vi "HovaCAL set params konfig.vi"(8 "Fehler (Eingang, kein Fehler)":errorcluster, 10 "Pump Idx":i32, 11 "TestKonfig (Eingang)":T1 {"TestKonfig Interferent"."Gasflasche MFC3" items=["----"=10000, "IAG NH3 3000"=0, "IAG NH3 200"=1, "IAG NH3 2000"=2, "IAG MG"=3, "IAG O2"=4]; "TestKonfig Interferent"."Gasflasche MFC2" items=["----"=10000, "IAG NH3 3000"=0, "IAG NH3 200"=1, "IAG NH3 2000"=2, "IAG MG"=3, "IAG O2"=4]; "TestKonfig Interferent"."Eingangs Konzentration MFC1" min=0.0; "TestKonfig Interferent"."Ausgangs Konzentration MFC1" min=0.0; "TestKonfig Interferent"."MFC2" items=["MFC 2", "MFC 3", "MFC 4", "MFC 5"]; "TestKonfig Interferent"."MFC3" items=["MFC 2", "MFC 3", "MFC 4", "MFC 5"]; "TestKonfig Interferent"."Ausgangs Konzentration MFC3" min=0.0; "TestKonfig Interferent"."Eingangs Konzentration MFC3" min=0.0; "TestKonfig Interferent"."Ausgangs Konzentration MFC2" min=0.0; "TestKonfig Interferent"."Eingangs Konzentration MFC2" min=0.0; "TestKonfig H2O"."HovaCAL Temperature" format="%.2f"; "TestKonfig H2O"."HovaCAL Flow Input Cluster"."HovaCAL Flow Input Cluster" format="%.2f"; "TestKonfig H2O"."Eingangs Konzentration:" min=0.0; "TestKonfig H2O"."zusätzliche Zeitdauer Erster Punkt" min=30 step=1 format="%#_5g"; "TestKonfig H2O"."Zeitdauer Stufen" format="%#_5g"; "TestKonfig H2O"."Max Fehler" format="%#_5g"; "TestKonfig H2O"."Anzahl Stufen" format="%#_5g"; "TestKonfig H2O"."Modus" items=["Messen", "CG zu Entnahmestelle"]}) -> (0 "Fehler (Ausgang)":errorcluster, 3 "TestKonfig (Ausgang)":T1 {"TestKonfig Interferent"."Gasflasche MFC3" items=["----"=10000, "IAG NH3 3000"=0, "IAG NH3 200"=1, "IAG NH3 2000"=2, "IAG MG"=3, "IAG O2"=4]; "TestKonfig Interferent"."Gasflasche MFC2" items=["----"=10000, "IAG NH3 3000"=0, "IAG NH3 200"=1, "IAG NH3 2000"=2, "IAG MG"=3, "IAG O2"=4]; "TestKonfig Interferent"."Eingangs Konzentration MFC1" min=0.0; "TestKonfig Interferent"."Ausgangs Konzentration MFC1" min=0.0; "TestKonfig Interferent"."MFC2" items=["MFC 2", "MFC 3", "MFC 4", "MFC 5"]; "TestKonfig Interferent"."MFC3" items=["MFC 2", "MFC 3", "MFC 4", "MFC 5"]; "TestKonfig Interferent"."Ausgangs Konzentration MFC3" min=0.0; "TestKonfig Interferent"."Eingangs Konzentration MFC3" min=0.0; "TestKonfig Interferent"."Ausgangs Konzentration MFC2" min=0.0; "TestKonfig Interferent"."Eingangs Konzentration MFC2" min=0.0; "TestKonfig H2O"."HovaCAL Temperature" format="%.2f"; "TestKonfig H2O"."HovaCAL Flow Input Cluster"."HovaCAL Flow Input Cluster" format="%.2f"; "TestKonfig H2O"."Eingangs Konzentration:" min=0.0; "TestKonfig H2O"."zusätzliche Zeitdauer Erster Punkt" min=30 step=1 format="%#_5g"; "TestKonfig H2O"."Zeitdauer Stufen" format="%#_5g"; "TestKonfig H2O"."Max Fehler" format="%#_5g"; "TestKonfig H2O"."Anzahl Stufen" format="%#_5g"; "TestKonfig H2O"."Modus" items=["Messen", "CG zu Entnahmestelle"]})   [LabVIEW 2020, in "EPA 1065.lvlib" / "HovaCAL Interference verificaton.lvlib"]
uses:
  HovaCAL Interference verificaton.lvlib
  TestKonfig.ctl
  TestKonfig H2O.ctl
  Modus.ctl
  Linearisierung V2/SpanEinstellungen/Einheit.ctl
  Linearisierung V2/Gasteiler/Stufen Tabelle 10 Stufen.ctl
  Linearisierung V2/Gasteiler/HovaCAL_Interface/Controls/Flow Einstellung.ctl
  Linearisierung V2/Gasteiler/HovaCAL_Interface/Controls/Temp Sollwerte Anzeige.ctl
  TestKonfig Interferents.ctl
  MFCAuswahl.ctl
  Seiten/System Einstellungen V2/Gasflasche Auswahl.ctl
  Linearisierung V2/Gasteiler/HovaCAL_Interface/Kommunikation/Aktion_FGV_HovaCAL_Interface_Kommunikation.ctl
  Linearisierung V2/Gasteiler/HovaCAL_Interface/Kommunikation/Aktion_FGV_HovaCAL_Interface_Kommandos.ctl
  Aktion Index uebersetzten.ctl
  Linearisierung V2/Gasteiler/HovaCAL_Interface/Kommunikation/Aktion_FGV_HovaCAL_Interface_SetData.ctl
  Linearisierung V2/Gasteiler/HovaCAL_Interface/Kommunikation/Kommunikation.lvlib
  Linearisierung V2/Gasteiler/Gasteiler.lvlib
  Linearisierung V2/SpanEinstellungen/SpanEinstellungen.lvlib
  Linearisierung V2/Gasteiler/HovaCAL_Interface/Controls/Controls.lvlib
  Seiten/System Einstellungen V2/System Einstellungen V2.lvlib
panel:
  # "sec"
  # "%"
  # "sec"
  # "sec"
  # "%"
  # "sec"
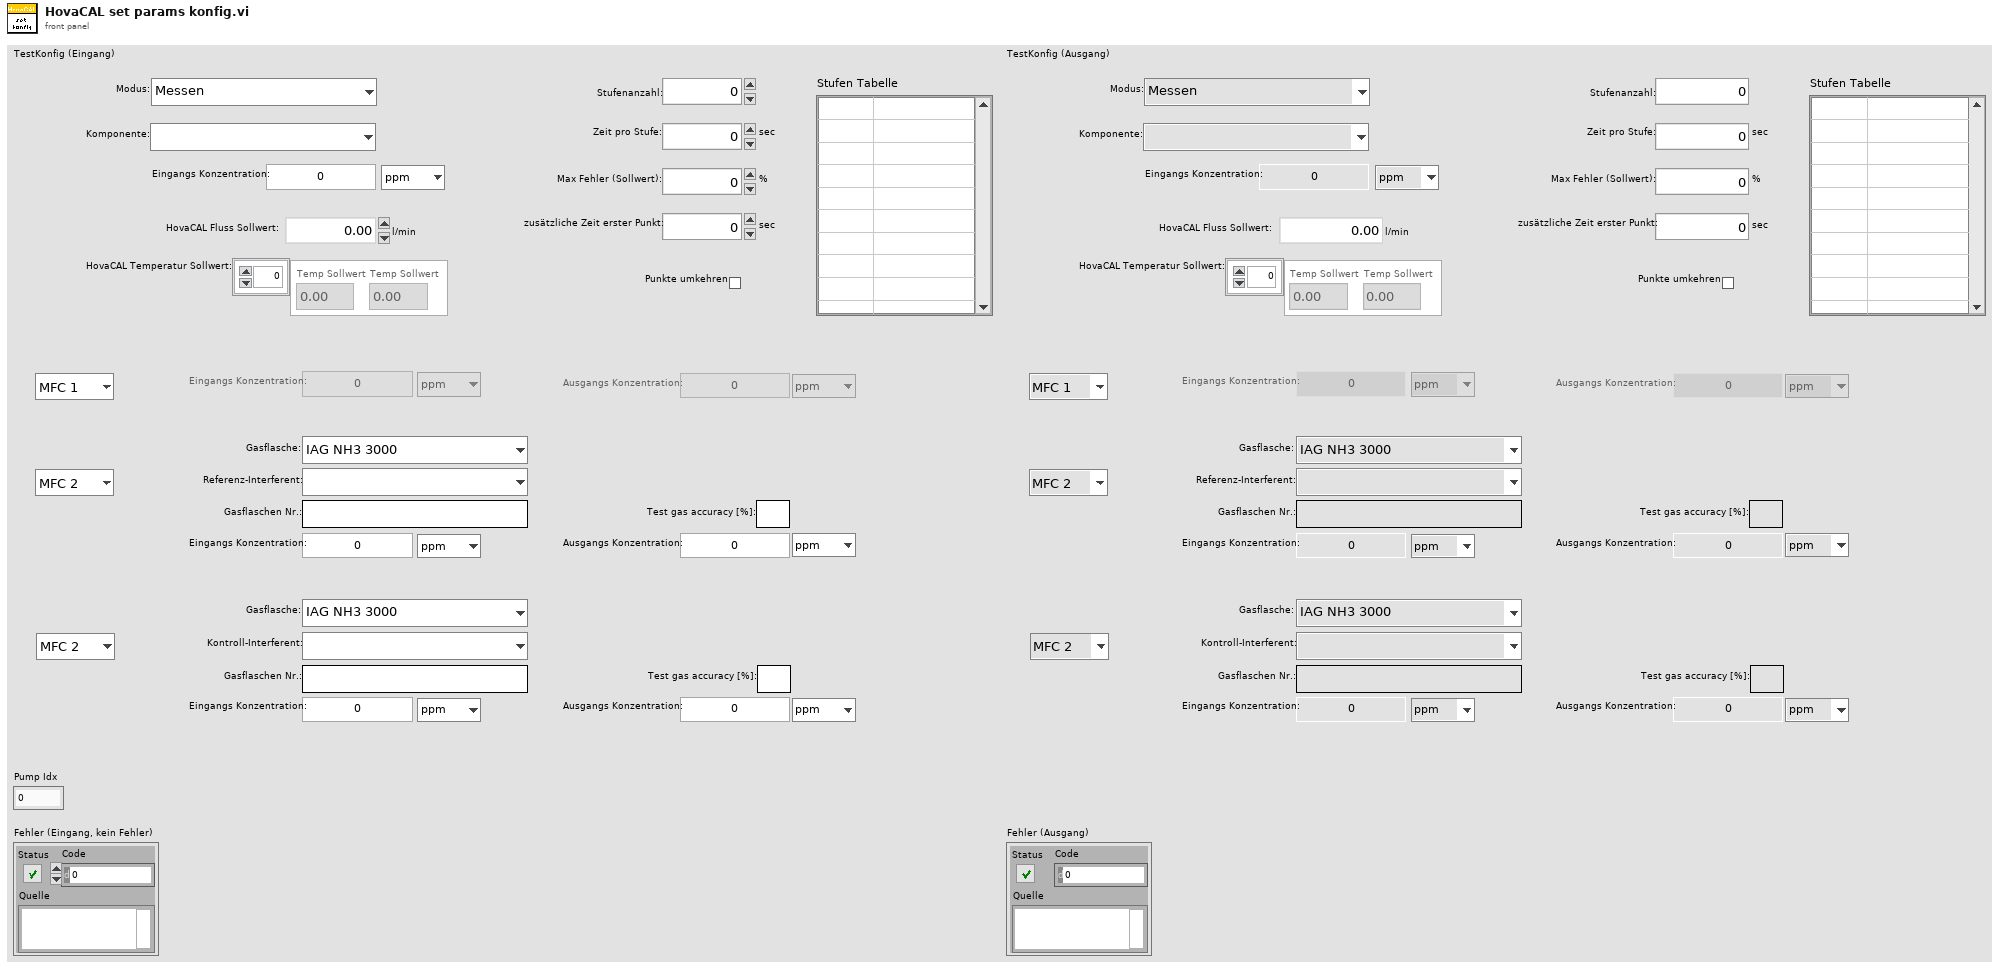
[diagram p1: front panel]
types:
  T1 = typedef "EPA 1065.lvlib/HovaCAL Interference verificaton.lvlib/TestKonfig.ctl" = cluster{"TestKonfig H2O":T2, "TestKonfig Interferent":T8}
  T2 = typedef "EPA 1065.lvlib/HovaCAL Interference verificaton.lvlib/TestKonfig H2O.ctl" = cluster{"Modus":T3, "Komponente:":u16, "Eingangs Konzentration:":dbl, "Einheit":T4, "Anzahl Stufen":sgl, "Zeitdauer Stufen":sgl, "Max Fehler":sgl, "zusätzliche Zeitdauer Erster Punkt":sgl, "Punkte umkehren":bool, "Stufen Tabelle":T5, "HovaCAL Flow Input Cluster":T6, "HovaCAL Temperature":T7}
  T3 = typedef "EPA 1065.lvlib/HovaCAL Interference verificaton.lvlib/Modus.ctl" = u16
  T4 = typedef "Linearisierung v2.lvlib/SpanEinstellungen.lvlib/Einheit.ctl" = enum16{"ppm", "%"}
  T5 = typedef "Linearisierung v2.lvlib/Gasteiler.lvlib/Stufen Tabelle 10 Stufen.ctl" = string[][]
  T6 = typedef "Linearisierung v2.lvlib/Gasteiler.lvlib/HovaCAL_Interface.lvlib/Controls.lvlib/Flow Einstellung.ctl" = cluster{"HovaCAL Flow Input Cluster":dbl}
  T7 = typedef "Linearisierung v2.lvlib/Gasteiler.lvlib/HovaCAL_Interface.lvlib/Controls.lvlib/Temp Sollwerte Anzeige.ctl" = dbl[]
  T8 = typedef "EPA 1065.lvlib/HovaCAL Interference verificaton.lvlib/TestKonfig Interferents.ctl" = cluster{"MFC1":enum16{"MFC 1"}, "Eingangs Konzentration MFC1":dbl, "Einheit MFC1 Eingang":T4, "Ausgangs Konzentration MFC1":dbl, "Einheit MFC1 Ausgang":T4, "MFC2":T9, "Referenz-Interferent:":u16, "Gasflaschen Nr MFC2":string, "Accuracy MFC2":string, "Eingangs Konzentration MFC2":dbl, "Einheit MFC2 Eingang":T4, "Ausgangs Konzentration MFC2":dbl, "Einheit MFC2 Ausgang":T4, "MFC3":T9, "Kontroll-Interferent:":u16, "Gasflaschen Nr MFC3":string, "Accuracy MFC3":string, "Eingangs Konzentration MFC3":dbl, "Einheit MFC3 Eingang":T4, "Ausgangs Konzentration MFC3":dbl, "Einheit MFC3 Ausgang":T4, "Gasflasche MFC2":T10, "Gasflasche MFC3":T10}
  T9 = typedef "EPA 1065.lvlib/HovaCAL Interference verificaton.lvlib/MFCAuswahl.ctl" = u16
  T10 = typedef "System Einstellungen V2.lvlib/Gasflasche Auswahl.ctl" = u16
  T11 = typedef "Linearisierung v2.lvlib/Gasteiler.lvlib/HovaCAL_Interface.lvlib/Kommunikation.lvlib/Aktion_FGV_HovaCAL_Interface_Kommunikation.ctl" = enum16{"Initialisieren", "Set Konzentrationen", "Set Gase", "Set Limits", "Get Dynamische Werte", "Beenden", "Com ändern", "Get Gase init", "Pause", "Get Gasteiler Infos", "Get MFC Infos", "Set Pumpen Parameter", "Set Pumpe Konzenration", "Set Pumpe run", "Set Temperaturen", "Set Fluss", "Get Gase", "Get Limits", "Get Dynamische Werte 1", "Get Dynamische Werte 2"}
  T12 = typedef "EPA 1065.lvlib/HovaCAL Interference verificaton.lvlib/Aktion Index uebersetzten.ctl" = enum16{"lesen", "schreiben", "auswerten", "Referenzwert", "KompIndex", "RefInterferIndex", "KontrInterfIndex"}
  T13 = typedef "Linearisierung v2.lvlib/Gasteiler.lvlib/HovaCAL_Interface.lvlib/Kommunikation.lvlib/Aktion_FGV_HovaCAL_Interface_Kommandos.ctl" = enum16{"lesen", "verarbeiten", "hinzufügen", "on top", "init", "sammeln", "freigeben", "connected"}
  T14 = typedef "String - Ausgabefeld.ctl" = string
  T15 = typedef "Linearisierung v2.lvlib/Gasteiler.lvlib/HovaCAL_Interface.lvlib/Kommunikation.lvlib/Aktion_FGV_HovaCAL_Interface_SetData.ctl" = enum16{"lesen", "Konzentrationen", "Pumpen Parameter", "Pumpe Konzentration", "Pumpe run", "Temperaturen", "Fluss", "Limits", "init"}
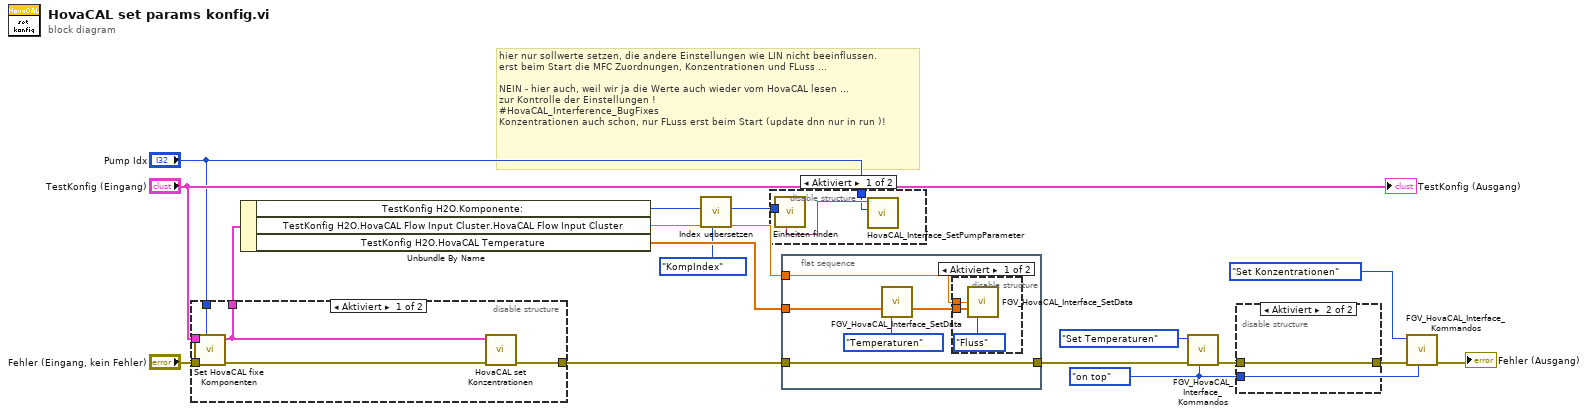
[diagram p0: block diagram]
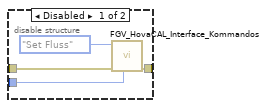
[diagram p2: hidden frame]
diagram:
  w5 = Aktion_FGV_HovaCAL_Interface_Kommandos."on top" ("Aktion")
  # "hier nur sollwerte setzen, die andere Einstellungen wie LIN nicht beeinflussen.\nerst beim Start die MFC Zuordnungen, Konzentrationen und FLuss ...\n\nNEIN - hier auch, weil wir ja die Werte auch wieder vom HovaCAL lesen ...\nzur Kontrolle der Einstellungen !\n#HovaCAL_Interference_BugFixes\nKonzentrationen auch schon, nur FLuss erst beim Start (update dnn nur in run )!"
  n1 = disable-structure shown="Aktiviert" {
    disable-tunnel: "Fehler (Eingang, kein Fehler)" -> [w23 w24]
    disable-tunnel: "TestKonfig (Eingang)" -> [w22 w25]
    disable-tunnel: "Pump Idx" -> [w21 _]
    disable-tunnel: [w20 w25] -> w6
    disable-tunnel: [w18 w24] -> w3
    frame Enabled {
      n2 = call "Set HovaCAL fixe Komponenten.vi"("Pump Idx"=w21, "Fehler (Eingang, kein Fehler)"=w23, "TestKonfig (Eingang)"=w22) -> ("Fehler (Ausgang)"=w19:errorcluster, "TestKonfig (Ausgang)"=w20:T1)  [unwired: 7 in]
      n3 = call "HovaCAL set Konzentrationen.vi"("Fehler (Eingang, kein Fehler)"=w19, "TestKonfig (Eingang)"=w20) -> ("Fehler (Ausgang)"=w18:errorcluster)  [unwired: 9 in]
    }
    frame Disabled {
    }
  }
  n4 = Unbundle By Name(w6) -> ("TestKonfig H2O.Komponente:"=w9:u16, "TestKonfig H2O.HovaCAL Flow Input Cluster.HovaCAL Flow Input Cluster"=w12:dbl, "TestKonfig H2O.HovaCAL Temperature"=w11:T7)
  n5 = call "Index uebersetzen.vi"("Aktion"=Aktion_Index_uebersetzten."KompIndex", "Index relativ:"=w9) -> ("Index absolut"=w8:i32)  [unwired: 4 in, 5 out]
  n6 = disable-structure shown="Aktiviert" {
    disable-tunnel: w8 -> [w27 _]
    disable-tunnel: "Pump Idx" -> [w26 _]
    frame Enabled {
      n7 = call "Einheiten finden.vi"("Komponente"=w27) -> ("Komponenten Name"=w28:T14)  [unwired: 6 in, 4 out]
      n8 = call "HovaCAL_Interface_SetPumpParameter.vi"("Pump Idx"=w26, "Komponent Name"=w28) -> ()  [unwired: 9 in, 1 out]
    }
    frame Disabled {
    }
  }
  n9 = flat-sequence {
    tunnel: w11 -> [w32]
    tunnel: w12 -> [w30]
    tunnel: w3 -> [w31]
    tunnel: [w31] -> w16
    frame #0 {
      n10 = call "FGV_HovaCAL_Interface_SetData.vi"("Temperature"=w32, "Aktion"=Aktion_FGV_HovaCAL_Interface_SetData."Temperaturen") -> ("Temperature out"=w29:dbl[])  [unwired: 7 in, 6 out]
      n11 = disable-structure shown="Aktiviert" {
        disable-tunnel: w30 -> [w35 _]
        disable-tunnel: w29 -> [w34 _]
        frame Enabled {
          n12 = call "FGV_HovaCAL_Interface_SetData.vi"("total flow setpoint in"=w35, "Temperature"=w34, "Aktion"=Aktion_FGV_HovaCAL_Interface_SetData."Fluss") -> ()  [unwired: 6 in, 7 out]
        }
        frame Disabled {
        }
      }
    }
  }
  n13 = call "FGV_HovaCAL_Interface_Kommandos.vi"("Aktion"=w5, "error in"=w16, "Kommando in"=Aktion_FGV_HovaCAL_Interface_Kommunikation."Set Temperaturen") -> ("error out"=w15:errorcluster)  [unwired: 2 in, 5 out]
  n14 = disable-structure shown="Aktiviert" {
    disable-tunnel: w15 -> [w40 w41]
    disable-tunnel: w5 -> [w38 _]
    disable-tunnel: [w37 w41] -> w1
    frame Disabled {
      n15 = call "FGV_HovaCAL_Interface_Kommandos.vi"("Aktion"=w38, "error in"=w40, "Kommando in"=Aktion_FGV_HovaCAL_Interface_Kommunikation."Set Fluss") -> ("error out"=w37:errorcluster)  [unwired: 2 in, 5 out]
    }
    frame Enabled {
    }
  }
  n16 = call "FGV_HovaCAL_Interface_Kommandos.vi"("Aktion"=w5, "error in"=w1, "Kommando in"=Aktion_FGV_HovaCAL_Interface_Kommunikation."Set Konzentrationen") -> ("error out"=→"Fehler (Ausgang)":errorcluster)  [unwired: 2 in, 5 out]
  "TestKonfig (Ausgang)" <- "TestKonfig (Eingang)"
